vi "Retrieve from DataBase.vi"(8 "error in (no error)":errorcluster, 10 "Search Criteria":string, 11 "DAO in":refnum<class "iDAO.lvclass">) -> (0 "error out":errorcluster, 3 "DAO out":refnum<class "iDAO.lvclass">)   [LabVIEW 2020, in "iDAO.lvclass"]
doc: "Retrieves all elements from the DataBase"
uses:
  iDAO.lvclass
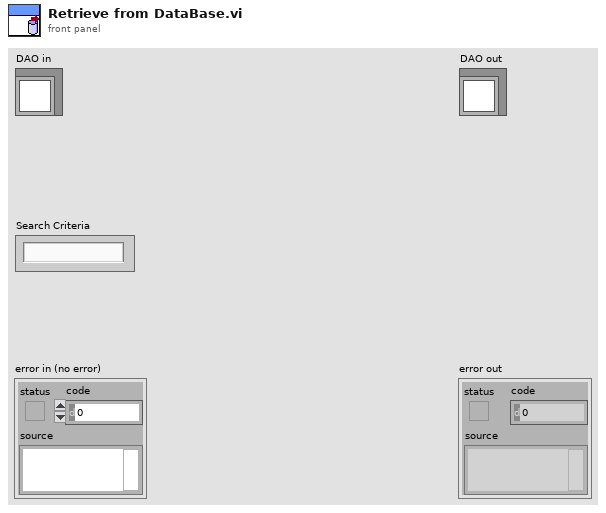
[diagram p1: front panel]
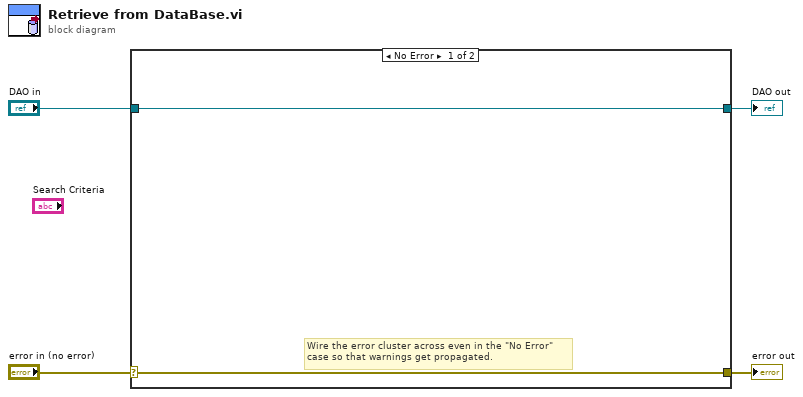
[diagram p0: block diagram]
diagram:
  n1 = case shown="No Error" "error in (no error)" {
    selector: "error in (no error)" -> [w5 w8]
    tunnel: [w5 w8] -> w3
    tunnel: [w6 w7] -> w1
    tunnel: "DAO in" -> [w6 w7]
    frame No Error {
      # "Wire the error cluster across even in the \"No Error\"\ncase so that warnings get propagated."
    }
    frame Error {
    }
  }
  "error out" <- w3
  "DAO out" <- w1
